vi "Math Test Suite (Result Event).vi"() -> ()   [LabVIEW 2013]
doc: "This example demonstrates how to programmatically save the test report to a file."
uses:
  classes/Test Result/Node Results.ctl
  classes/Test Result/Test Node.ctl
  classes/Test Result/Test Registration Data.ctl
  classes/Test Result/Assert Event Data.ctl
  classes/Test Result/Test Result.lvclass
  classes/Test Suite/Test Suite.lvclass
panel:
  out "Extended Results received":bool
  out "Test Logs":string
  out "Test failed":bool
  out "assert-update-event":string
  out "assert-event":string
  out "test-event":string
  out "Legacy Results received":bool
  out "Suite Results Event":T1[](array[typedef])
  out "Returned Results":T1[](array[typedef])
  out "Test Suite Error Output":errorcluster
  # "See block diagram"
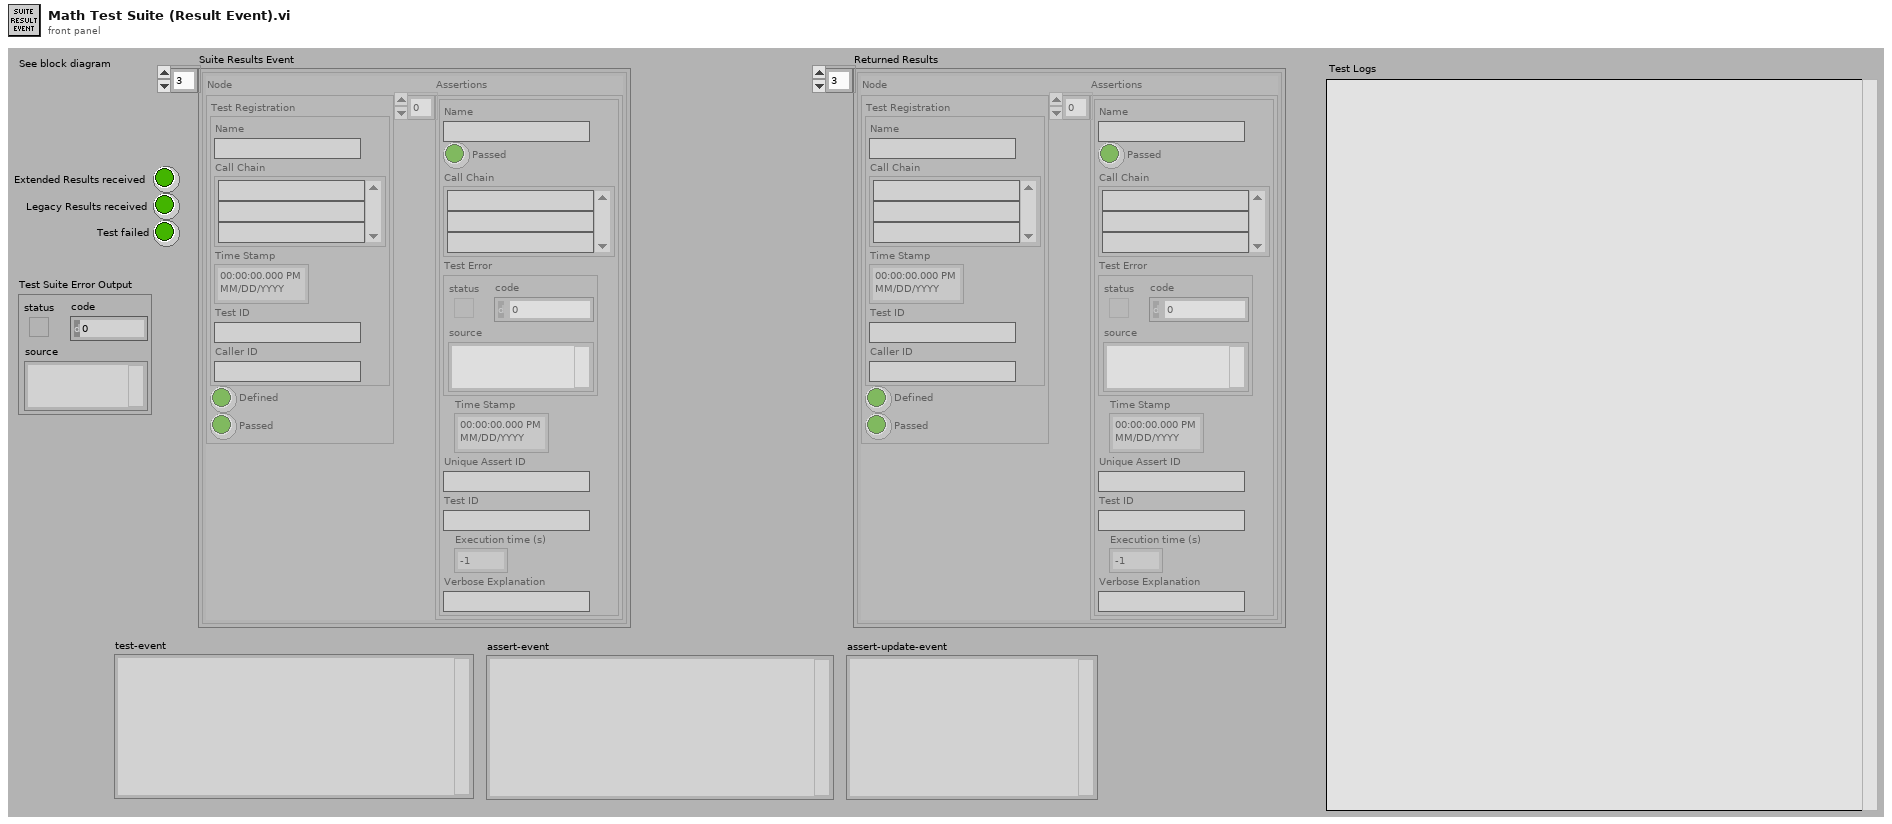
[diagram p1: front panel]
types:
  T1 = typedef "Caraya.lvlib/Test Result.lvclass/Node Results.ctl" = cluster{"Node":T2, "Assertions":T4[]}
  T2 = typedef "Caraya.lvlib/Test Result.lvclass/Test Node.ctl" = cluster{"Test Registration":T3, "Defined":bool, "Passed":bool}
  T3 = typedef "Caraya.lvlib/Test Result.lvclass/Test Registration Data.ctl" = cluster{"Name":string, "Call Chain":string[], "Time Stamp":timestamp, "Test ID":string, "Caller ID":string}
  T4 = typedef "Caraya.lvlib/Test Result.lvclass/Assert Event Data.ctl" = cluster{"Name":string, "Passed":bool, "Call Chain":string[], "Test Error":errorcluster, "Time Stamp":timestamp, "Unique Assert ID":string, "Test ID":string, "Execution time (s)":dbl, "Verbose Explanation":string}
  T5 = typedef "Caraya.lvlib/Test Suite.lvclass/Suite PublicEvents -- cluster.ctl" = cluster{"Test Suite Result Event":refnum<user-event>, "suite destroyed":refnum<user-event>, "Test Registration Event":refnum<user-event>, "Assertion Event":refnum<user-event>, "Assertion Update Event":refnum<user-event>}
  T6 = typedef "Caraya.lvlib/Test Result.lvclass/Node Results (Extended).ctl" = cluster{"Test Node":T7, "Assertions":T8[]}
  T7 = typedef "Caraya.lvlib/Test Result.lvclass/Test Node (Extended).ctl" = cluster{"Test Registration":T3, "Defined":bool, "Passed":bool, "properties":variant}
  T8 = typedef "Caraya.lvlib/Test Result.lvclass/Assert Event Data (Extended).ctl" = cluster{"name":string, "passed":bool, "call-chain":string[], "test-error":errorcluster, "timestamp":timestamp, "assert-id":string, "test-id":string, "time":dbl, "message":string, "properties":variant, "measurements":variant, "user-defined":variant}
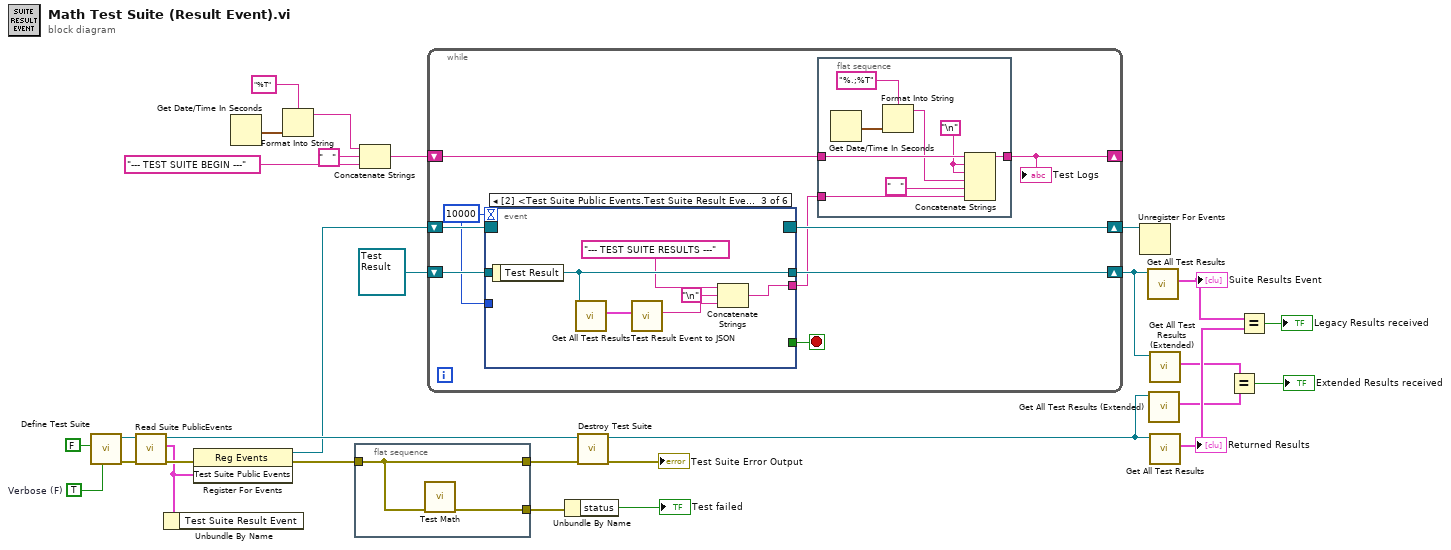
[diagram p0: block diagram]
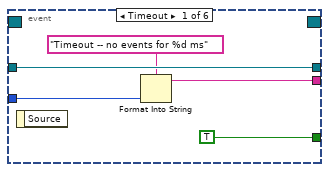
[diagram p2: hidden frame]
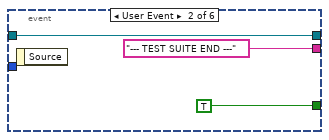
[diagram p3: hidden frame]
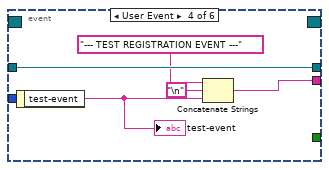
[diagram p4: hidden frame]
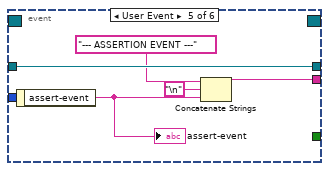
[diagram p5: hidden frame]
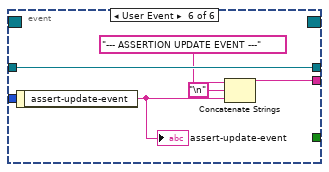
[diagram p6: hidden frame]
diagram:
  w28 = TRUE  # Verbose (F)
  n1 = call "Define Test Suite.vi"("Verbose (F)"=w28, "Interactive"=FALSE) -> ("error out"=w27:errorcluster, "Test Suite"=w26:refnum<class "Test Suite.lvclass">)  [unwired: 7 in, 1 out]
  n2 = call "Read Suite PublicEvents.vi"("error in (no error)"=w27, "Test Suite in"=w26) -> ("error out"=w24:errorcluster, "Test Suite Public Events"=w1:T5, "Test Suite out"=w25:refnum<class "Test Suite.lvclass">)  [unwired: 7 in]
  n3 = Unbundle By Name(w1) -> ()  [unwired: 1 out]
  n4 = register-events(error in=w24, w1) -> (reference out=w23:refnum<event-registration>, error out=w15:errorcluster)  [unwired: 1 in]
  n5 = Get Date/Time In Seconds() -> (seconds since 1Jan1904=w11:timestamp)
  n6 = Format Into String(format string="%T", w11) -> (resulting string=w10:string)  [unwired: 2 in, 1 out]
  n7 = flat-sequence {
    tunnel: [w31] -> w16
    tunnel: w15 -> [w31]
    tunnel: [w30] -> w14
    frame #0 {
      n8 = call "Test Math.vi"("error in (no error)"=w31) -> ("error out"=w30:errorcluster)  [unwired: 10 in]
    }
  }
  n9 = Concatenate Strings(w10, "   " ("format string"), "--- TEST SUITE BEGIN ---" ("format string")) -> (w7:string)
  n10 = while {
    shift-right: [w38] -> w6
    shift-left: refnum<class "Test Result.lvclass"> refnum ("Test Result") -> [w37]
    shift-right: [w34] -> _
    shift-left: w7 -> [w35]
    shift-right: [w39] -> w21
    shift-left: w23 -> [w40]
    stop <- w36 stop-if-true
    w33 = 10000
    n11 = event shown="[2] <Test Suite Public Events.Test Suite Result Event>: User Event" {
      selector: w40 -> [_ _ _ _ _ _]
      dyn-events: [_ _ _ _ _ _] -> w39
      timeout: w33 -> [_ _ _ _ _ _]
      tunnel: [w53 w56 w62 w67 w72 w77] -> w38
      tunnel: w37 -> [w53 w56 _ w67 w72 w77]
      tunnel: [TRUE TRUE _ _ _ _] -> w36
      tunnel: [w49 "--- TEST SUITE END ---" w57 w63 w68 w74] -> w32
      tunnel: w33 -> [w51 _ _ _ _ _]
      event Timeout {
        n12 = event-data() -> ()  [unwired: 1 in, 1 out]
        n13 = Format Into String(format string="Timeout -- no events for %d ms" ("assert-update-event"), w51) -> (resulting string=w49:string)  [unwired: 2 in, 1 out]
      }
      event User Event {
        n14 = event-data() -> ()  [unwired: 1 in, 1 out]
      }
      event User Event {
        n15 = event-data() -> ("Test Result"=w62:refnum<class "Test Result.lvclass">)  [unwired: 1 in]
        n16 = call "Get All Test Results.vi"("Test Result in"=w62) -> ("Test Results"=w61:T1[])  [unwired: 8 in, 2 out]
        n17 = call "Test Result Event to JSON.vi"("Test Results Event"=w61) -> ("<JSON>Test Results Event"=w59:string)  [unwired: 10 in]
        n18 = Concatenate Strings("--- TEST SUITE RESULTS ---", "\n", w59) -> (w57:string)
      }
      event User Event {
        n19 = event-data() -> ("test-event"=w64:string)  [unwired: 1 in]
        "test-event" <- w64
        n20 = Concatenate Strings("--- TEST REGISTRATION EVENT ---", "\n", w64) -> (w63:string)
      }
      event User Event {
        n21 = event-data() -> ("assert-event"=w69:string)  [unwired: 1 in]
        "assert-event" <- w69
        n22 = Concatenate Strings("--- ASSERTION EVENT ---", "\n", w69) -> (w68:string)
      }
      event User Event {
        n23 = event-data() -> ("assert-update-event"=w73:string)  [unwired: 1 in]
        "assert-update-event" <- w73
        n24 = Concatenate Strings("--- ASSERTION UPDATE EVENT ---", "\n", w73) -> (w74:string)
      }
    }
    n25 = flat-sequence {
      tunnel: w35 -> [w48]
      tunnel: [w47] -> w34
      tunnel: w32 -> [w44]
      frame #0 {
        w43 = "\n"
        n26 = Get Date/Time In Seconds() -> (seconds since 1Jan1904=w46:timestamp)
        n27 = Format Into String(format string="%.;%T", w46) -> (resulting string=w45:string)  [unwired: 2 in, 1 out]
        n28 = Concatenate Strings(w48, w43, w43, w45, "   " ("format string"), w44) -> (w47:string)
      }
    }
    "Test Logs" <- w34
  }
  n29 = Unbundle By Name(w14) -> ("status"=→"Test failed":bool)
  n30 = call-dynamic "Destroy Test Suite.vi"("error in (no error)"=w16, "Test Suite in"=w25) -> ("error out"=→"Test Suite Error Output":errorcluster, "Test Suite Results"=w5:refnum<class "Test Result.lvclass">)  [unwired: 8 in]
  n31 = Unregister For Events(event registration refnum=w21) -> ()  [unwired: 1 in, 1 out]
  n32 = call "Get All Test Results.vi"("Test Result in"=w6) -> ("Test Results"=w20:T1[])  [unwired: 8 in, 2 out]
  "Suite Results Event" <- w20
  n33 = call "Get All Test Results (Extended).vi"("Test Result in"=w5) -> ("Test Results"=w3:T6[])  [unwired: 8 in, 2 out]
  n34 = call "Get All Test Results (Extended).vi"("Test Result in"=w6) -> ("Test Results"=w4:T6[])  [unwired: 8 in, 2 out]
  n35 = call "Get All Test Results.vi"("Test Result in"=w5) -> ("Test Results"=w19:T1[])  [unwired: 8 in, 2 out]
  "Returned Results" <- w19
  n36 = Equal?(x=w4, y=w3) -> (x = y?=→"Extended Results received":bool)
  n37 = Equal?(x=w20, y=w19) -> (x = y?=→"Legacy Results received":bool)
